vi "F to C.vi"(11 "Slide":i64) -> (3 "Numeric":dbl)   [LabVIEW 2024]
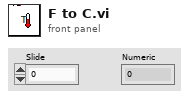
[diagram p1: front panel]
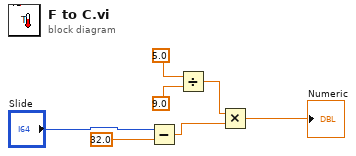
[diagram p0: block diagram]
diagram:
  n1 = Subtract(x="Slide", y=32.0) -> (x-y=w4:dbl)
  n2 = Divide(x=5.0, y=9.0) -> (x/y=w5:dbl)
  n3 = Multiply(x=w5, y=w4) -> (x*y=→"Numeric":dbl)
